vi "Do.vi"(8 "error in (no error)":errorcluster, 10 "Actor in":refnum<class "Actor.lvclass">, 11 "Configure TV Trigger Source [TV] Msg":refnum<class "Configure TV Trigger Source [TV] Msg.lvclass">) -> (0 "error out":errorcluster, 2 "Actor out":refnum<class "Actor.lvclass">)   [LabVIEW 2014, in "CS++Scope.lvlib" / "Configure TV Trigger Source [TV] Msg.lvclass"]
doc: "This VI delivers the message to the actor by calling the appropriate method(s) on the actor."
uses:
  Configure TV Trigger Source [TV] Msg.lvclass
  <vilib>/ActorFramework/Actor/Actor.lvclass
  CS++Scope/CS++Scope.lvclass
  Configure TV Trigger Source [TV] Msg.lvclass/Configure TV Trigger Source [TV] Msg.ctl
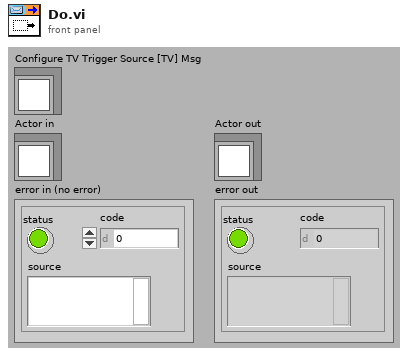
[diagram p1: front panel]
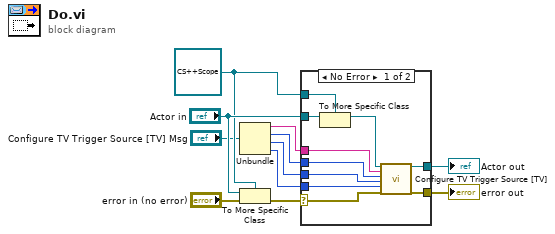
[diagram p0: block diagram]
diagram:
  w6 = refnum<class "CS++Scope.lvclass"> refnum ("Actor in")
  n1 = Unbundle ("Main-Unbundle")("Configure TV Trigger Source [TV] Msg") -> (w4:string, w3:i32, w2:i32, w1:i32)
  n2 = To More Specific Class(target class=w6, reference="Actor in", error in="error in (no error)") -> (error out=w10:errorcluster)  [unwired: 1 out]
  n3 = case shown="No Error" w10 {
    selector: w10 -> [w19 w23]
    tunnel: [w21 w23] -> w9
    tunnel: [w20 w22] -> w8
    tunnel: "Actor in" -> [w18 w22]
    tunnel: w6 -> [w17 _]
    tunnel: w4 -> [w15 _]
    tunnel: w3 -> [w14 _]
    tunnel: w2 -> [w13 _]
    tunnel: w1 -> [w12 _]
    frame No Error {
      n4 = To More Specific Class(target class=w17, reference=w18) -> (specific class reference=w16:refnum<class "CS++Scope.lvclass">)  [unwired: 1 in, 1 out]
      n5 = call "Configure TV Trigger Source [TV].vi"("CS++Scope"=w16, "trigger source (\"CHANNEL1\")"=w15, "tv event (Field 1)"=w14, "tv trigger polarity (Positive)"=w13, "tv signal format (NTSC)"=w12, "error in (no error)"=w19) -> ("CS++Scope out"=w20:refnum<class "CS++Scope.lvclass">, "error out"=w21:errorcluster)  [unwired: 12 in]
    }
    frame Error {
    }
  }
  "error out" <- w9
  "Actor out" <- w8
